vi "Served_Global.vi"(0 "Mode":T1) -> (1 "Served VI Name":string[](array[string]), 2 "Served VI Path":path[](array[path]), 3 "Served IP Number & Port No":string[](array[string]))   [LabVIEW 2010]
uses:
  Controls/Serveds.ctl
  Constants_global.vi
  Preference_global.vi
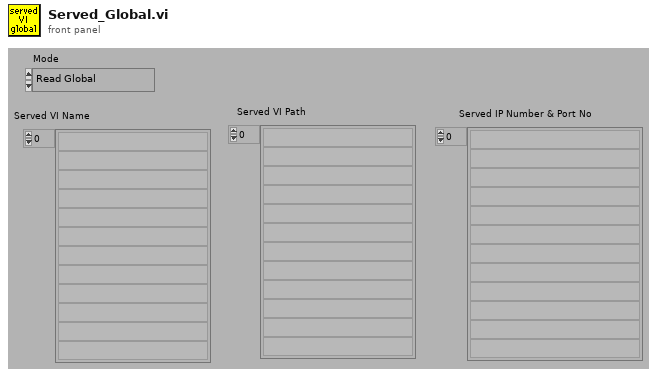
[diagram p1: front panel]
types:
  T1 = typedef "Serveds.ctl" = enum16{"Read Global", "Load Global From File"}
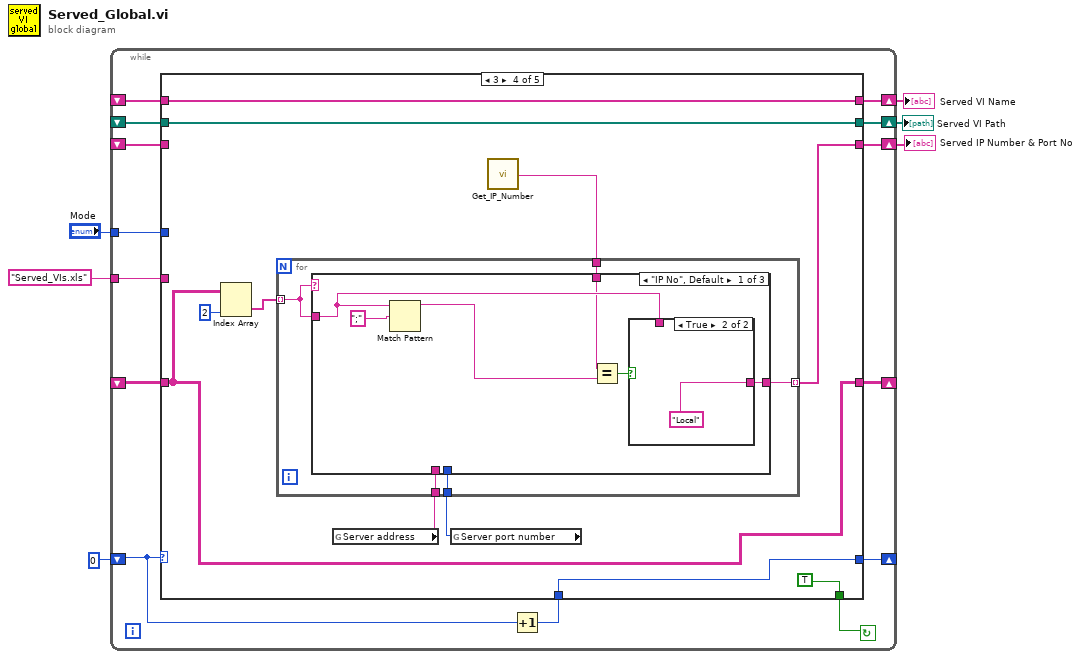
[diagram p0: block diagram]
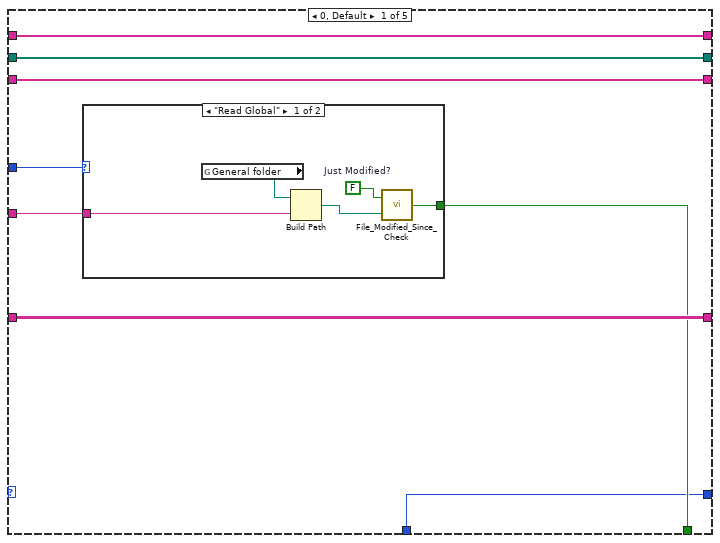
[diagram p2: hidden frame]
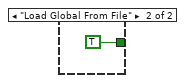
[diagram p3: hidden frame]
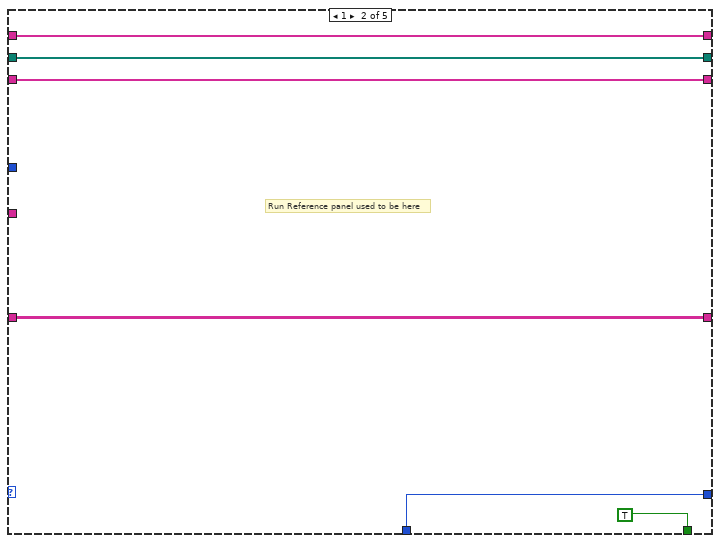
[diagram p4: hidden frame]
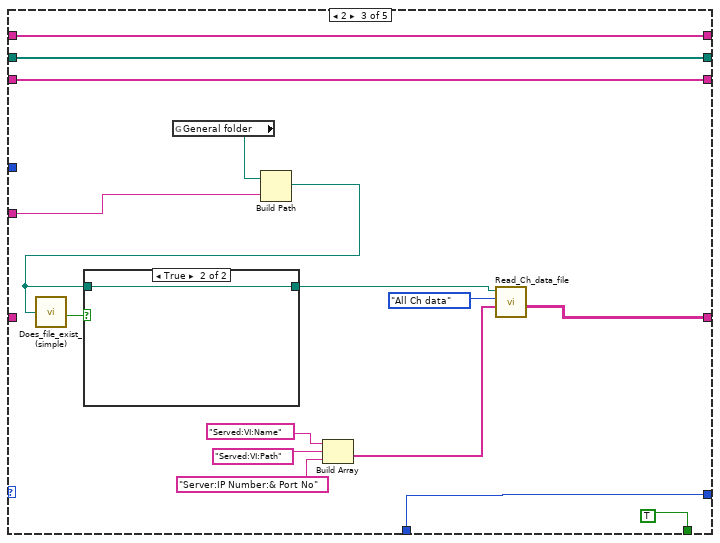
[diagram p5: hidden frame]
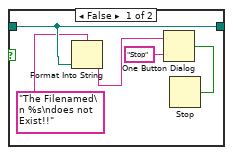
[diagram p6: hidden frame]
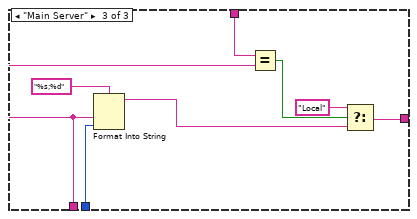
[diagram p9: hidden frame]
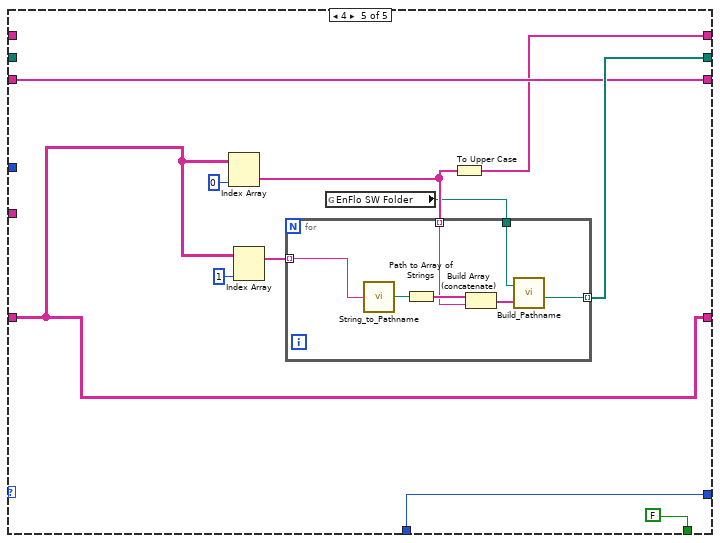
[diagram p10: hidden frame]
diagram:
  n1 = while {
    shift-left: _ -> [w8]
    shift-right: [w13] -> w4
    shift-left: _ -> [w12]
    shift-right: [w11] -> w3
    shift-left: _ -> [w10]
    shift-right: [w9] -> w2
    shift-left: _ -> [w16]
    shift-right: [w17] -> _
    tunnel: "Mode" -> [w18]
    shift-left: 0 -> [w15]
    shift-right: [w19] -> _
    tunnel: "Served_VIs.xls" ("Substring") -> [w7]
    stop <- w20 continue-if-true
    n2 = Increment(x=w15) -> (x+1=w14:i32)
    n3 = case shown="3" w15 {
      tunnel: [w26 TRUE TRUE TRUE FALSE] -> w20
      tunnel: [w25 w38 w49 w70 w105] -> w19
      tunnel: w18 -> [w27 _ _ _ _]
      tunnel: [w28 w40 w54 w67 w99] -> w17
      tunnel: w16 -> [w28 w40 _ w67 w99]
      tunnel: w14 -> [w25 w38 w49 w70 w105]
      tunnel: [w22 w35 w42 w68 w101] -> w13
      tunnel: w12 -> [w23 w36 w43 w65 _]
      tunnel: [w23 w36 w43 w65 w102] -> w11
      tunnel: w10 -> [w24 w37 w44 w64 _]
      tunnel: [w24 w37 w44 w64 w96] -> w9
      tunnel: w8 -> [w22 w35 w42 _ w101]
      tunnel: w7 -> [w21 _ w41 _ _]
      frame 0, Default {
        n4 = case shown="\"Read Global\"" w27 {
          tunnel: [w31 TRUE ("Modified?")] -> w26
          tunnel: w21 -> [w29 _]
          frame "Read Global" {
            w30 = FALSE  # Just Modified?
            n5 = global read "Constants_global.vi" "General folder"() -> (w33:path)
            n6 = Build Path(base path=w33, name or relative path=w29) -> (appended path=w32:path)
            n7 = call "File_Modified_Since_Check.vi"("Pathname"=w32, "Just Modified?"=w30) -> ("Modified?"=w31:bool)
          }
          frame "Load Global From File" {
          }
        }
      }
      frame 1 {
        # "Run Reference panel used to be here"
      }
      frame 2 {
        n8 = global read "Constants_global.vi" "General folder"() -> (w53:path)
        n9 = Build Path(base path=w53, name or relative path=w41) -> (appended path=w50:path)
        n10 = call "Does_file_exist_(simple).vi"("Pathname"=w50) -> ("exists?"=w52:bool)
        n11 = case shown="True" w52 {
          tunnel: w50 -> [w58 w62]
          tunnel: [w58 w62] -> w51
          frame False {
            n12 = Format Into String(format string="The Filenamed\n %s\ndoes not Exist!!" ("Format String"), w58) -> (resulting string=w60:string)  [unwired: 2 in, 1 out]
            n13 = One Button Dialog(message=w60, button name ("OK")="Stop") -> (true=w59:bool)
            n14 = Stop(stop? (T)=w59) -> ()
          }
          frame True {
          }
        }
        n15 = Build Array("Served:VI:Name", "Served:VI:Path", "Server:IP Number:& Port No") -> (w45:string[])
        n16 = call "Read_Ch_data_file.vi"("Present Channels"=w45, "Output"=enum16{"All Ch data", "The last few rows"}."All Ch data", "Filename"=w51) -> ("Channel Values"=w54:string[][])  [unwired: 2 in, 4 out]
      }
      frame 3 {
        n17 = Index Array(array=w67, index (col)=2) -> (element=w66:string[])  [unwired: 1 in]
        n18 = global read "Preference_global.vi" "Server address"() -> (w72:string)
        n19 = global read "Preference_global.vi" "Server port number"() -> (w71:u32)
        n20 = call "Get_IP_Number.vi"() -> ("IP Number"=w63:string)
        n21 = for {
          tunnel: [w78] -> w68 mode=indexing
          tunnel: w72 -> [w77]
          tunnel: w71 -> [w76]
          tunnel: w63 -> [w75]
          tunnel: w66 -> [w74] mode=indexing
          n22 = case shown="\"IP No\", Default" w74 {
            tunnel: [w83 w87 w88] -> w78
            tunnel: w77 -> [_ _ w92]
            tunnel: w76 -> [_ _ w95]
            tunnel: w74 -> [w81 w87 _]
            tunnel: w75 -> [w79 _ w93]
            frame "IP No", Default {
              n23 = Match Pattern(string=w81, regular expression=";") -> (before substring=w80:string)  [unwired: 4 out]
              n24 = Equal?(x=w79, y=w80) -> (x = y?=w82:bool)
              n25 = case shown="True" w82 {
                tunnel: [w85 "Local" ("t")] -> w83
                tunnel: w81 -> [w85 _]
                frame False {
                }
                frame True {
                }
              }
            }
            frame "Local" {
            }
            frame "Main Server" {
              n26 = Format Into String(format string="%s;%d" ("Format String"), w92, w95) -> (resulting string=w90:string)  [unwired: 2 in, 1 out]
              n27 = Equal?(x=w93, y=w92) -> (x = y?=w91:bool)
              n28 = Select(t="Local", s=w91, f=w90) -> (s? t:f=w88:string)
            }
          }
        }
      }
      frame 4 {
        n29 = Index Array(array=w99, index (col)=0 ("Index")) -> (element=w98:string[])  [unwired: 1 in]
        n30 = Index Array(array=w99, index (col)=1 ("Index")) -> (element=w103:string[])  [unwired: 1 in]
        n31 = global read "Constants_global.vi" "EnFlo SW Folder"() -> (w97:path)
        n32 = for {
          tunnel: w103 -> [w113] mode=indexing
          tunnel: [w107] -> w102 mode=indexing
          tunnel: w98 -> [w110] mode=indexing
          tunnel: w97 -> [w109]
          n33 = call "String_to_Pathname.vi"("Input String"=w113) -> ("path"=w112:path)
          n34 = Path to Array of Strings(0:w112) -> (2:w111:string[])  [unwired: 1 out]
          n35 = Build Array (concatenate)(w111, w110) -> (w108:string[])
          n36 = call "Build_Pathname.vi"("Output Array"=w108, "Pathname"=w109) -> ("Appended path"=w107:path)
        }
        n37 = To Upper Case(1:w98) -> (0:w96:string[])
      }
    }
  }
  "Served IP Number & Port No" <- w4
  "Served VI Name" <- w2
  "Served VI Path" <- w3
